vi "MDAQ_CalibrationCalc.vi"() -> ()   [LabVIEW 2021]
uses:
  <vilib>/Analysis/NI_AALPro.lvlib
  <vilib>/Analysis/NI_AAL_SigProc.lvlib
  GUI_Def.ctl
  Status_Cluster.ctl
panel:
  out "x*y":dbl
  in  "Numeric":dbl
  in  "Status_Cluster Out":T1 {"GATESTOP" format="%04x"; "GATESTRT" format="%04x"; "AMPLITUDE" format="%04x"; "M_CYCLES" format="%04x"; "N_CYCLES" format="%04x"; "STEP" format="%04x"; "BASE" format="%04x"; "CHAN" format="%04x"}
  in  "Fit Select":bool
  out "Calibrated Graph":cluster{dbl, u32}[](graph)
  out "Mirror Fit":T2
  out "Fit":T2
  out "Plot":cluster{dbl[], dbl[]}[](graph)
  out "XY Graph":cluster{cluster{dbl, dbl}[]}[](graph)
  out "Waveform Graph":u32[](graph)
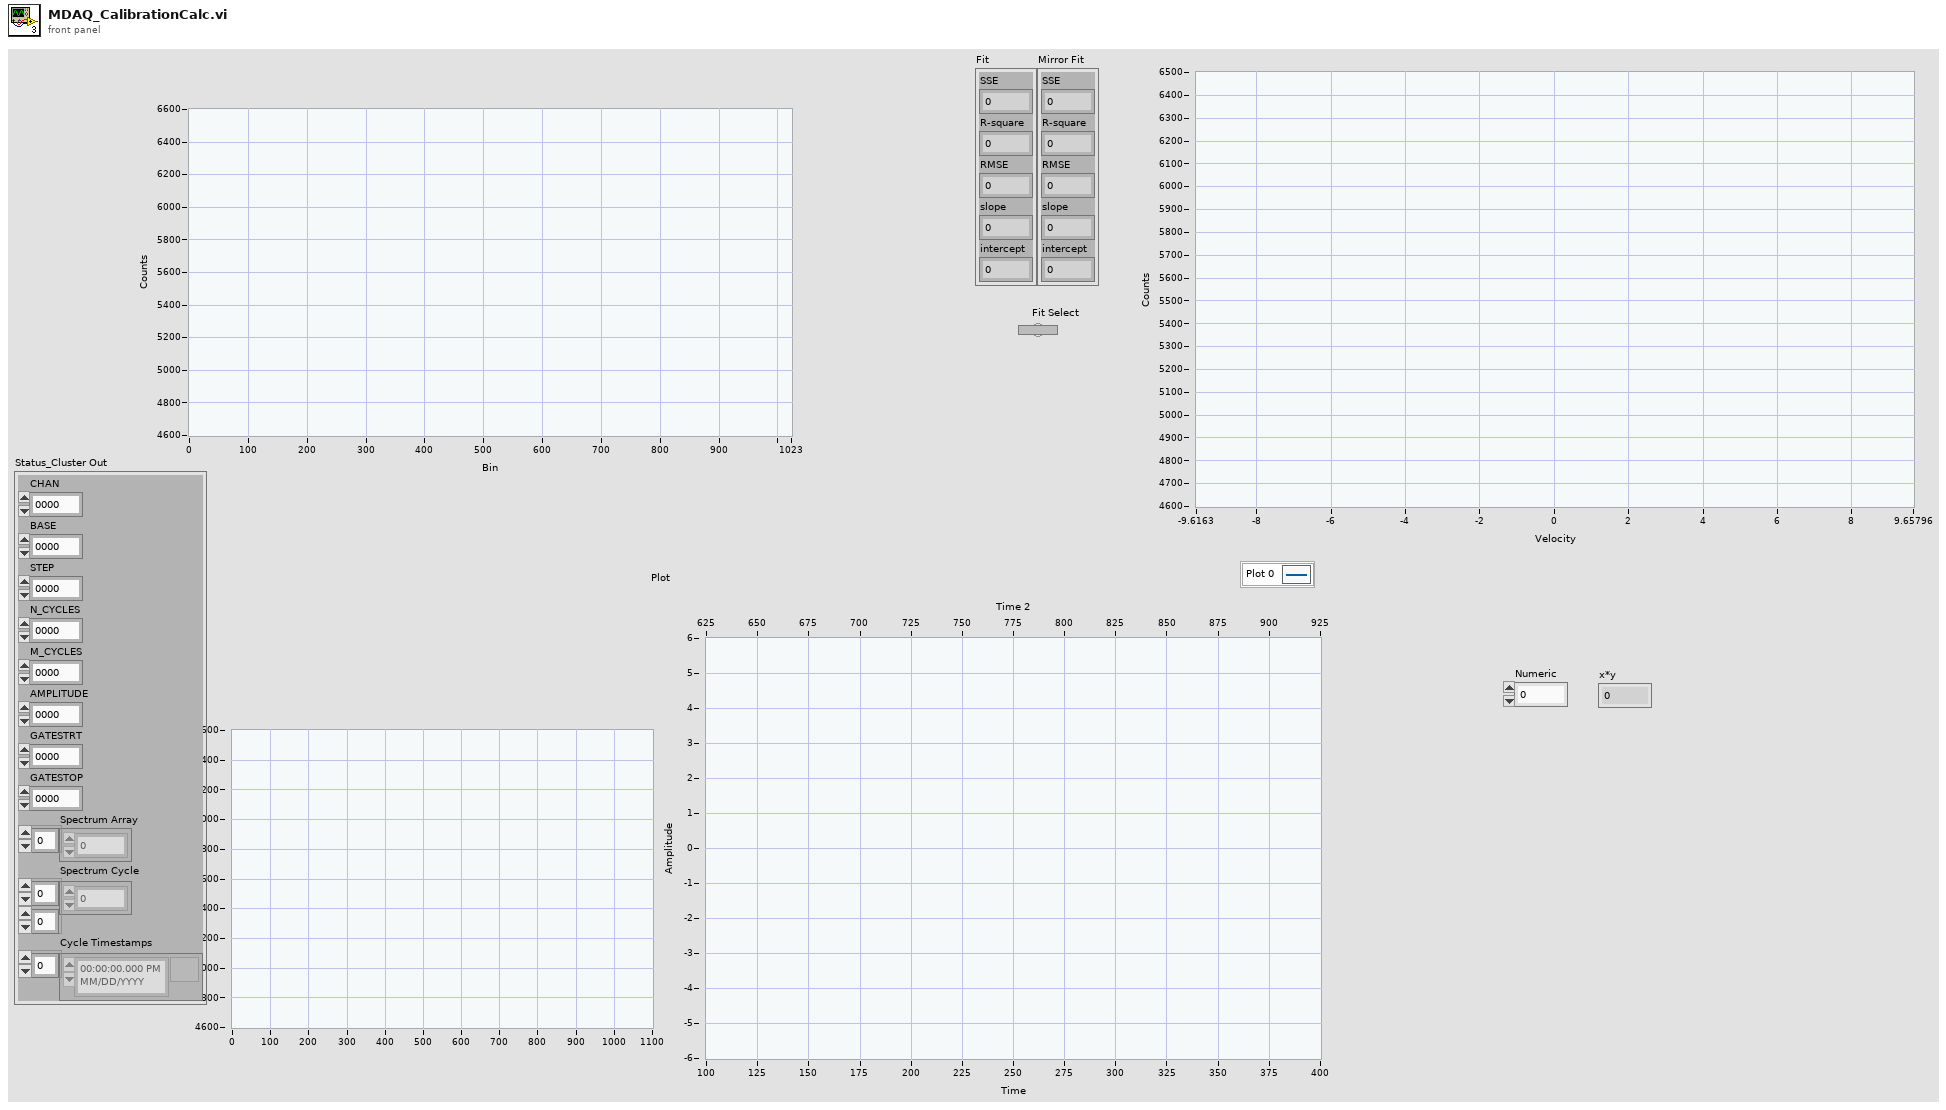
[diagram p1: front panel]
types:
  T1 = typedef "Status_Cluster.ctl" = cluster{"CHAN":u32, "BASE":u32, "STEP":u32, "N_CYCLES":u32, "M_CYCLES":u32, "AMPLITUDE":u32, "GATESTRT":u32, "GATESTOP":u32, "Spectrum Array":u32[], "Spectrum Cycle":u32[][], "Cycle Timestamps":timestamp[]}
  T2 = cluster{"SSE":dbl, "R-square":dbl, "RMSE":dbl, "slope":dbl, "intercept":dbl}
  T3 = typedef "GUI_Def.ctl" = cluster{"Monitor MSG":string, "Request Read":bool, "Cycle TimeStamp":timestamp, "CV":cluster{"Set Point Index":u32, "Run Start TimeS":timestamp, "Last SP Index":u32, "No. Set Points":u32, "Target Set Points":dbl[], "CV Data Array":cluster{"Counts Array":cluster{timestamp, i32}[]}[], "CV Normalised Array":cluster{"Counts Array":cluster{timestamp, dbl}[]}[], "Reverse?":bool, "NormalizationFactor":i32[], "CycleNo":i32, "SurfaceCV":dbl[][], "New Cycle":bool}, "Normal":cluster{"Collecting":bool}, "Getting Mode":enum16{"Off", "Normal", "CV"}}
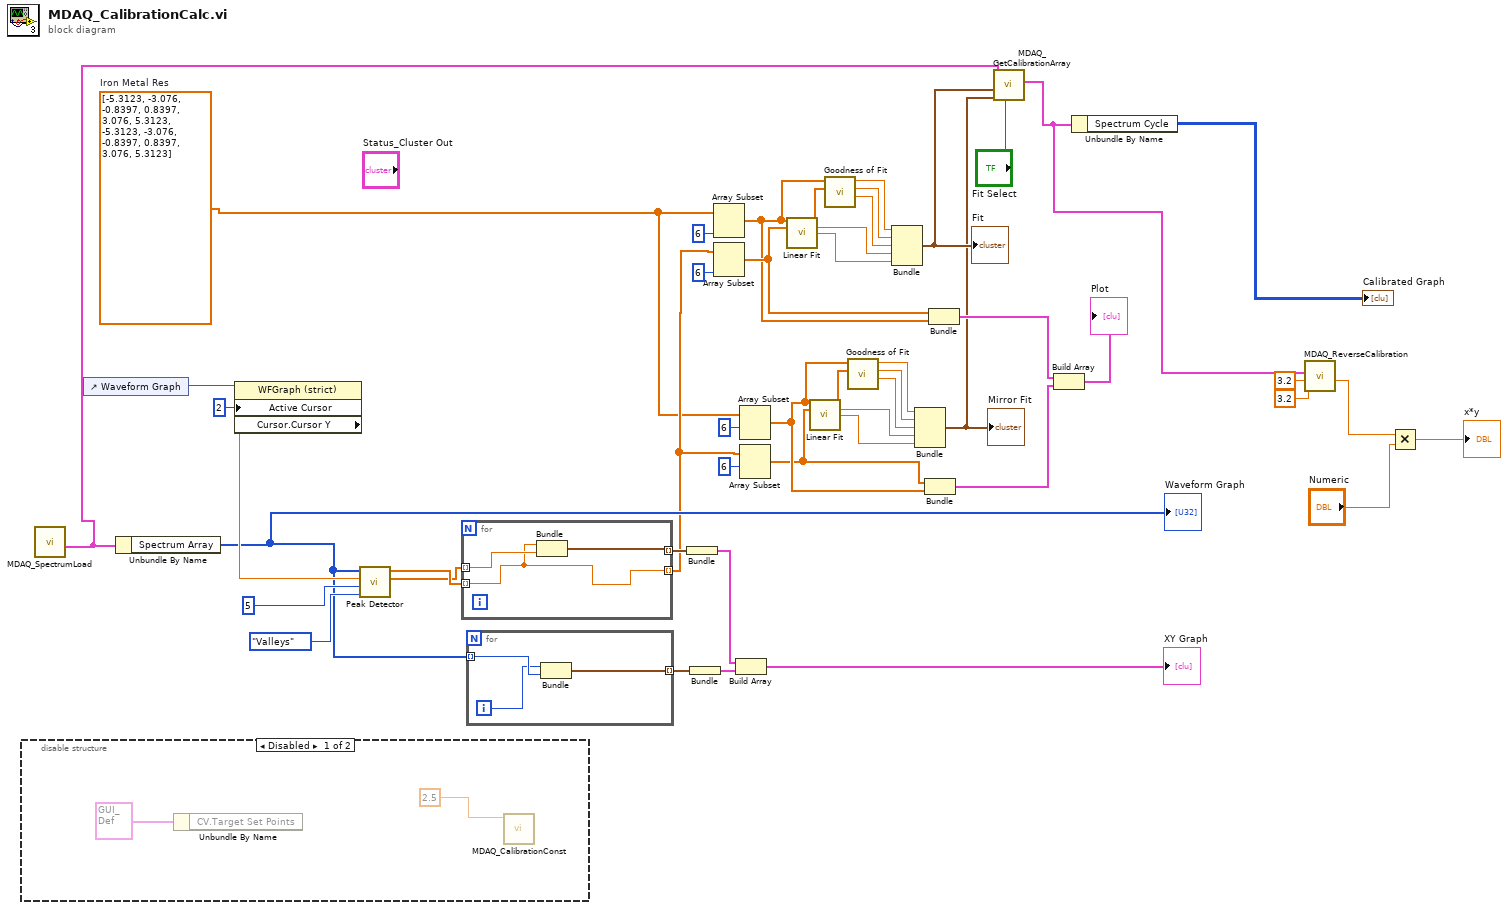
[diagram p0: block diagram]
diagram:
  w31 = dbl[] [-5.3123, -3.076, -0.8397, 0.8397, 3.076, 5.3123, -5.3123, -3.076, -0.8397, 0.8397, 3.076, 5.3123]  # Iron Metal Res
  n1 = disable-structure shown="Disabled" {
    frame Disabled {
      n2 = Unbundle By Name(T3 {"Monitor MSG"="", "Request Read"=FALSE, "Cycle TimeStamp"=timestamp(0 s since 1904-01-01), "CV"={"Set Point Index"=0, "Run Start TimeS"=timestamp(0 s since 1904-01-01), "Last SP Index"=0, "No. Set Points"=0, "Target Set Points"=[], "CV Data Array"=[], "CV Normalised Array"=[], "Reverse?"=FALSE, "NormalizationFactor"=[], "CycleNo"=0, "SurfaceCV"=[], "New Cycle"=FALSE}, "Normal"={"Collecting"=FALSE}, "Getting Mode"=enum."Off"}) -> ()  [unwired: 1 out]
      n3 = call "MDAQ_CalibrationConst.vi"("MDU Velocity"=2.5) -> ()  [unwired: 10 in, 1 out]
    }
    frame Enabled {
    }
  }
  n4 = call "MDAQ_SpectrumLoad.vi"() -> ("Status_Cluster Out"=w11:T1)  [unwired: 10 in, 1 out]
  n5 = control-ref of="Waveform Graph"() -> (w49:refnum<vi>)
  n6 = Unbundle By Name(w11) -> ("Spectrum Array"=w38:u32[])
  "Waveform Graph" <- w38
  n7 = property class="WFGraph (strict)"(reference=w49, "Active Cursor"=u32 2) -> ("Cursor.Cursor Y"=w47:dbl)  [unwired: 1 in, 2 out]
  n8 = call <vilib>:"Peak Detector.vi"("peaks/valleys"=enum32{"Peaks", "Valleys"}."Valleys", "width"=5, "threshold"=w47, "X"=w38) -> ("Amplitudes"=w43:dbl[], "Locations"=w44:dbl[])  [unwired: 3 in, 3 out]
  n9 = for {
    tunnel: w44 -> [w52] mode=indexing
    tunnel: [w52] -> w32 mode=indexing
    tunnel: w43 -> [w53] mode=indexing
    tunnel: [w54] -> w42 mode=indexing
    n10 = Bundle(w52, w53) -> (w54:cluster{dbl, dbl})  [unwired: 1 in]
  }
  n11 = for {
    tunnel: w38 -> [w57] mode=indexing
    tunnel: [w55] -> w41 mode=indexing
    i -> [w56]
    n12 = Bundle(w56, w57) -> (w55:cluster{i32, u32})  [unwired: 1 in]
  }
  n13 = Bundle(w42) -> (w40:cluster{cluster{dbl, dbl}[]})  [unwired: 1 in]
  n14 = Bundle(w41) -> (w39:cluster{cluster{i32, u32}[]})  [unwired: 1 in]
  n15 = Array Subset(array=w31, length=6) -> (w26:dbl[])  [unwired: 1 in]
  n16 = Array Subset(array=w32, length=6) -> (w30:dbl[])  [unwired: 1 in]
  n17 = Build Array(w40, w39) -> (→"XY Graph":cluster{cluster{dbl, dbl}[]}[])
  n18 = Array Subset(array=w31, index=6) -> (w13:dbl[])  [unwired: 1 in]
  n19 = Array Subset(array=w32, index=6) -> (w12:dbl[])  [unwired: 1 in]
  n20 = call <vilib>:"Linear Fit.vi"("Y"=w26, "X"=w30) -> ("Best Linear Fit"=w25:dbl[], "slope"=w21:dbl, "intercept"=w20:dbl)  [unwired: 9 in, 2 out]
  n21 = call <vilib>:"Linear Fit.vi"("Y"=w13, "X"=w12) -> ("Best Linear Fit"=w19:dbl[], "slope"=w15:dbl, "intercept"=w14:dbl)  [unwired: 9 in, 2 out]
  n22 = call <vilib>:"Goodness of Fit.vi"("Best Fit"=w25, "Y"=w26) -> ("RMSE"=w22:dbl, "R-square"=w23:dbl, "SSE"=w24:dbl)  [unwired: 6 in, 1 out]
  n23 = call <vilib>:"Goodness of Fit.vi"("Best Fit"=w19, "Y"=w13) -> ("RMSE"=w16:dbl, "R-square"=w17:dbl, "SSE"=w18:dbl)  [unwired: 6 in, 1 out]
  n24 = Bundle("SSE"=w24, "R-square"=w23, "RMSE"=w22, "slope"=w21, "intercept"=w20) -> (w10:T2)  [unwired: 1 in]
  "Fit" <- w10
  n25 = Bundle("SSE"=w18, "R-square"=w17, "RMSE"=w16, "slope"=w15, "intercept"=w14) -> (w9:T2)  [unwired: 1 in]
  "Mirror Fit" <- w9
  n26 = Bundle(w12, w13) -> (w27:cluster{dbl[], dbl[]})  [unwired: 1 in]
  n27 = Bundle(w30, w26) -> (w29:cluster{dbl[], dbl[]})  [unwired: 1 in]
  n28 = call "MDAQ_GetCalibrationArray.vi"("Fit Select"="Fit Select", "Mirror Fit"=w9, "Fit"=w10, "Cluster In"=w11) -> ("Cluster Out"=w6:T1)  [unwired: 7 in]
  n29 = Build Array(w29, w27) -> (→"Plot":cluster{dbl[], dbl[]}[])
  n30 = Unbundle By Name(w6) -> ("Spectrum Cycle"=→"Calibrated Graph":u32[][])
  n31 = call "MDAQ_ReverseCalibration.vi"("MDU Velocity"=3.2, "MDAQ Calibration"=3.2, "Main Cluster in"=w6) -> ("Scaler"=w2:dbl)  [unwired: 7 in, 1 out]
  n32 = Multiply(x=w2, y="Numeric") -> (x*y=→"x*y":dbl)
